vi "Autonomous Independent.vi"() -> ()   [LabVIEW 2016]
doc: "This VI is called when autonomous begins, and will automatically be terminated when autonomous ends. You can carry out timed or sensor driven robot movement independently without needing to return to the caller."
uses:
  Refname/Huskie Board.ctl
  Refname/Refname to String (Huskie Board).vi
  Robot Global Data.vi
panel:
  in  "error in":errorcluster
  out "error out":errorcluster
  # "Be sure to right-click and choose Data Operations>>Make Current Value default if you want to save the array values with the VI"
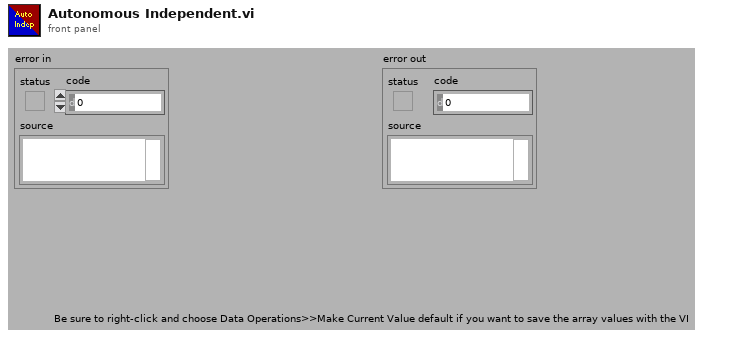
[diagram p1: front panel]
types:
  T1 = typedef "Huskie Board.ctl" = enum16{"Huskie Board", "Log Queue", ""}
  T2 = typedef "WPI_SerialPortRef.ctl" = cluster{"DevStatus":errorcluster, "Serial Port Name":refnum<visa-resource-name>}
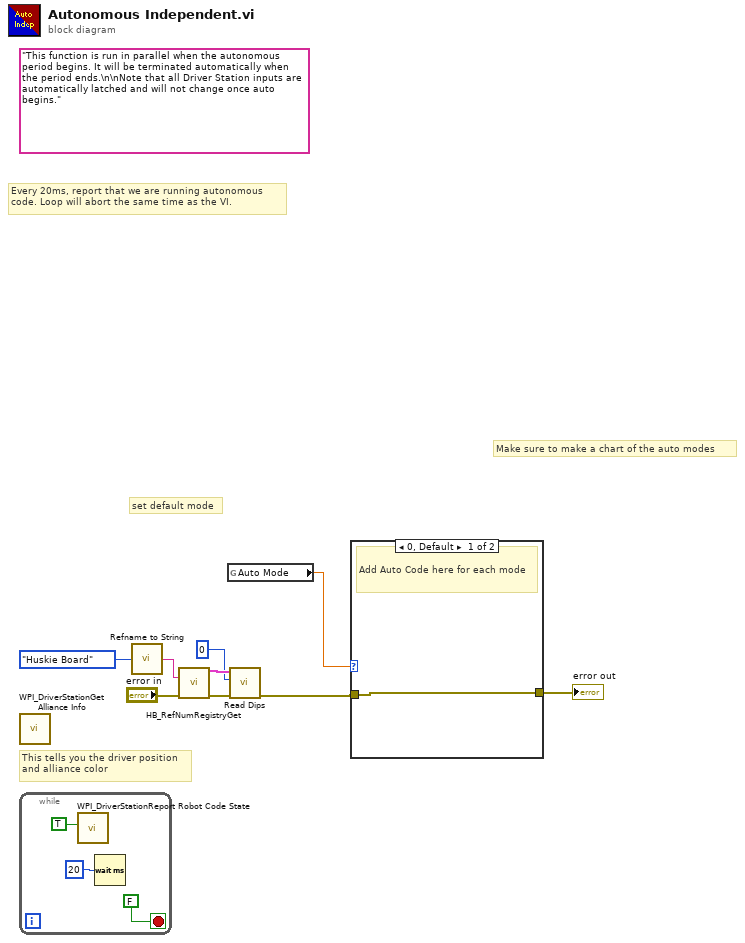
[diagram p0: block diagram]
diagram:
  (unwired) "This function is run in parallel when the autonomous period begins. It will be terminated automatically when the period ends.\n\nNote that all Driver Station inputs are automatically latched and will not change once auto begins."
  # "Make sure to make a chart of the auto modes"
  # "set default mode"
  # "Every 20ms, report that we are running autonomous\ncode. Loop will abort the same time as the VI."
  # "This tells you the driver position\nand alliance color"
  n1 = call <vilib>:"WPI_DriverStationGet Alliance Info.vi"() -> ()  [unwired: 12 out]
  n2 = while {
    stop <- FALSE stop-if-true
    n3 = call <vilib>:"WPI_DriverStationReport Robot Code State.vi"("Autonomous"=TRUE) -> ()  [unwired: 10 in, 1 out]
    n4 = Wait (ms)(milliseconds to wait=u32 20) -> ()  [unwired: 1 out]
  }
  n5 = call-poly "Refname to String.vi"("Enum"=Huskie_Board."Huskie Board") -> ("resulting string"=w8:string)
  n6 = call <vilib>:"HB_RefNumRegistryGet.vi"("refnum name"=w8, "error in (no error)"="error in") -> ("HBDevRef"=w6:T2, "error out"=w5:errorcluster)  [unwired: 12 in]
  n7 = global read "Robot Global Data.vi" "Auto Mode"() -> (w2:dbl)
  n8 = call "Read Dips.vi"("error in"=w5, "Default"=0, "HBDevRef"=w6) -> ("error out"=w3:errorcluster)  [unwired: 8 in]
  n9 = case shown="0, Default" w2 {
    tunnel: w3 -> [w13 w14]
    tunnel: [w13 w14] -> w1
    frame 0, Default {
      # "Add Auto Code here for each mode"
    }
    frame 1 {
    }
  }
  "error out" <- w1
